vi "setCommandEvents.vi"(8 "error in (no error)":errorcluster, 10 "Tools.lvlib:Interpreters.lvlib:CommandEvents.lvclass":refnum<class "CommandEvents.lvclass">, 11 "CommandProcessor.lvclass in":refnum<class "CommandProcessor.lvclass">) -> (0 "error out":errorcluster, 3 "CommandProcessor.lvclass out":refnum<class "CommandProcessor.lvclass">)   [LabVIEW 2011, in "Tools.lvlib" / "Interpreters.lvlib" / "CommandProcessor.lvclass"]
uses:
  CommandProcessor.lvclass
  CommandEvents/CommandEvents.lvclass
  CommandProcessor.lvclass/CommandProcessor.ctl
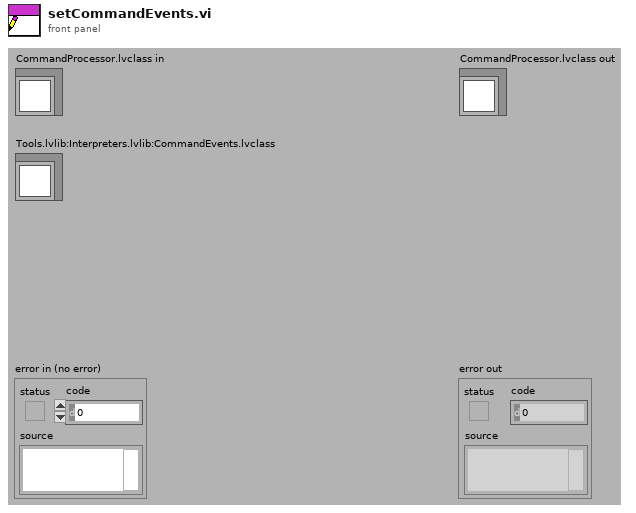
[diagram p1: front panel]
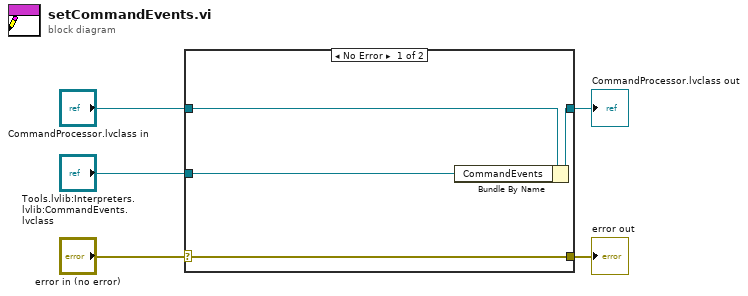
[diagram p0: block diagram]
diagram:
  n1 = case shown="No Error" "error in (no error)" {
    selector: "error in (no error)" -> [w9 w10]
    tunnel: [w9 w10] -> w4
    tunnel: [w7 w11] -> w2
    tunnel: "CommandProcessor.lvclass in" -> [w8 w11]
    tunnel: "Tools.lvlib:Interpreters.lvlib:CommandEvents.lvclass" -> [w6 _]
    frame No Error {
      n2 = Bundle By Name(cluster=w8, "CommandEvents"=w6) -> (w7:refnum<class "CommandProcessor.lvclass">)
    }
    frame Error {
    }
  }
  "error out" <- w4
  "CommandProcessor.lvclass out" <- w2
